vi "HandleError.vi"(6 "error-status":u8, 8 "Error In":errorcluster, 9 "Error String":string) -> (0 "Error Out":errorcluster)   [LabVIEW 2018, in "SensorPlugins.lvlib" / "RoomAlert.lvclass"]
doc: "Formats the string and numeric values and merges it into the error clustor."
uses:
  RoomAlert.lvclass
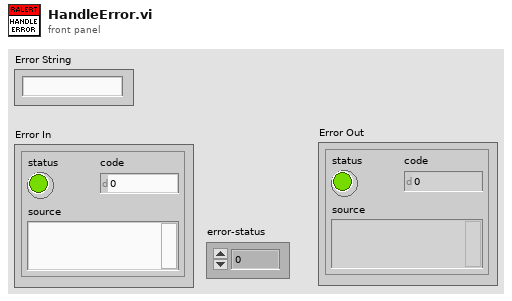
[diagram p1: front panel]
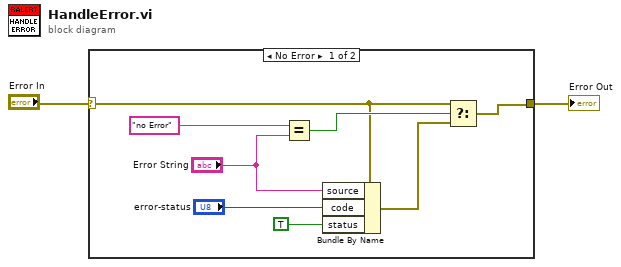
[diagram p0: block diagram]
diagram:
  n1 = case shown="No Error" "Error In" {
    selector: "Error In" -> [w4 w11]
    tunnel: [w3 w11] -> w1
    frame No Error {
      n2 = Equal?(x="no Error" ("error-string"), y="Error String") -> (x = y?=w9:bool)
      n3 = Bundle By Name(cluster=w4, "source"="Error String", "code"="error-status", "status"=TRUE) -> (w5:errorcluster)
      n4 = Select(t=w4, s=w9, f=w5) -> (s? t:f=w3:errorcluster)
    }
    frame Error {
    }
  }
  "Error Out" <- w1
